vi "ZBX Control Example.vi"() -> ()   [LabVIEW 2023]
uses:
  <instrlib>/niUSRP/Reference FPGA/ZBX Control/ATR state.ctl
  <vilib>/Platform/TimedLoop/XDataNode/wakeup.ctl
  <vilib>/Platform/TimedLoop/XDataNode/XDNodeRunTimeDep.lvlib
  <vilib>/Platform/TimedLoop/XDataNode/nitl_modes.ctl
  <vilib>/Platform/TimedLoop/XDataNode/timing_clust.ctl
  <vilib>/Platform/TimedLoop/XDataNode/XDataNode.xnode
panel:
  in  "TX samples":u64
  in  "RX samples":u64
  in  "rx gain high":u32
  in  "rx gain low":u32
  in  "tx gain":u32
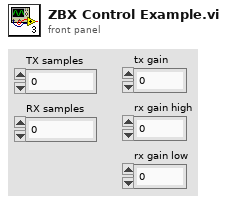
[diagram p1: front panel]
types:
  T1 = typedef "XDNodeRunTimeDep.lvlib/timing_clust.ctl" = cluster{"Expected End [f-1]":u64, "Actual End [f-1]":u64, "Finished Late? [f-1]":bool, "Expected End [i-1]":u64, "Actual End [i-1]":u64, "Finished Late? [i-1]":bool, "Expected Start [i]":u64, "Actual Start [i]":u64, "Expected Start [f]":u64, "Actual Start [f]":u64, "Source Name":string, "Structure Name":string, "Period":i64, "Deadline":i64, "Offset":i64, "Start":i64, "Priority":i32, "Timeout":i32, "Mode":T2, "Wakeup Reason":T3, "Error":errorcluster, "Source Type":string, "Secondary Source Type":string, "Global End Time":u64, "Global Start Time":u64, "Frame Duration":u64, "Iteration Duration":u64, "Assigned CPU":i32, "I/O Scan Engine Mode":u32}
  T2 = typedef "XDNodeRunTimeDep.lvlib/nitl_modes.ctl" = enum32{"No Change", "Process missed periods, maintain original phase", "Discard missed periods, maintain original phase", "Process missed periods, ignore original phase", "Discard missed periods, ignore original phase"}
  T3 = typedef "XDNodeRunTimeDep.lvlib/wakeup.ctl" = enum32{"Normal", "Aborted", "Asynchronous wakeup", "Timing source error", "Timed loop error", "Timeout"}
  T4 = typedef "ATR state.ctl" = enum8{"Idle", "RX", "TX", "TRX"}
  T5 = typedef "ZBX IO Response.ctl" = cluster{"response Ack":bool, "response data":u32, "response status":fxp<+,2,2>}
  T6 = typedef "ZBX IO Request.ctl" = cluster{"I/O Address":fxp<+,20,20>, "I/O Request Data":u32, "request write":bool, "request read":bool, "request has time":bool, "request time":u64}
  T7 = typedef "Dboard IOs.ctl" = cluster{"CtrlPortReqAddr":refnum<k21>, "CtrlPortReqData":refnum<k21>, "CtrlPortReqWr":refnum<k21>, "CtrlPortReqRd":refnum<k21>, "CtrlPortReqHasTime":refnum<k21>, "CtrlPortReqTime":refnum<k21>, "CtrlPortRespAck":refnum<k21>, "CtrlPortRespData":refnum<k21>, "CtrlPortRespStatus":refnum<k21>}
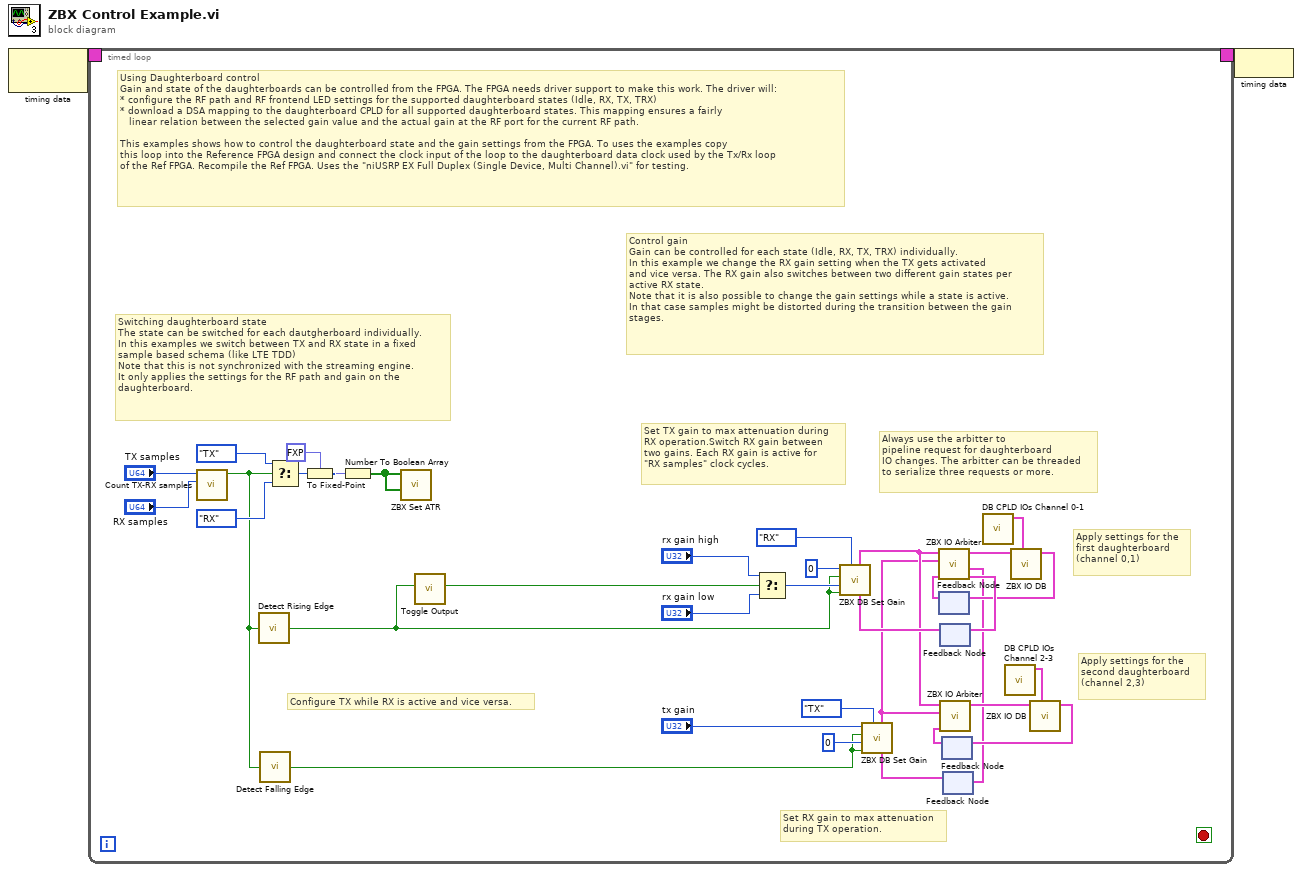
[diagram p0: block diagram]
diagram:
  n1 = node-c288() -> (w2:T1)  [unwired: 1 in]
  n2 = timed-loop {
    timing: w2 -> [_]
    timing-out: [_] -> w1
    stop <- _ stop-if-true
    # "Configure TX while RX is active and vice versa."
    # "Set RX gain to max attenuation\nduring TX operation."
    # "Set TX gain to max attenuation during\nRX operation.Switch RX gain between\ntwo gains. Each RX gain is active for\n\"RX samples\" clock cycles."
    # "Using Daughterboard control\nGain and state of the daughterboards can be controlled from the FPGA. The FPGA needs driver support to make this work. The driver will:\n* configure the RF path and RF frontend LED settings for the supported daughterboard states (Idle, RX, TX, TRX)\n* download a DSA mapping to the daughterboard CPLD for all supported daughterboard states. This mapping ensures a fairly \n   linear relation between the selected gain value and the actual gain at the RF port for the current RF path.\n\nThis examples shows how to control the daughterboard state and the gain settings from the FPGA. To uses the examples copy\nthis loop into the Reference FPGA design and connect the clock input of the loop to the daughterboard data clock used by the Tx/Rx loop\nof the Ref FPGA. Recompile the Ref FPGA. Uses the \"niUSRP EX Full Duplex (Single Device, Multi Channel).vi\" for testing."
    # "Always use the arbitter to\npipeline request for daughterboard\nIO changes. The arbitter can be threaded\nto serialize three requests or more."
    # "Apply settings for the\nsecond daughterboard \n(channel 2,3)"
    # "Apply settings for the\nfirst daughterboard \n(channel 0,1)"
    # "Control gain\nGain can be controlled for each state (Idle, RX, TX, TRX) individually.\nIn this example we change the RX gain setting when the TX gets activated\nand vice versa. The RX gain also switches between two different gain states per\nactive RX state.\nNote that it is also possible to change the gain settings while a state is active.\nIn that case samples might be distorted during the transition between the gain\nstages."
    # "Switching daughterboard state\nThe state can be switched for each dautgherboard individually.\nIn this examples we switch between TX and RX state in a fixed\nsample based schema (like LTE TDD)\nNote that this is not synchronized with the streaming engine. \nIt only applies the settings for the RF path and gain on the \ndaughterboard."
    n3 = call <instrlib>:"Count TX-RX samples.vi"("RX samples"="RX samples", "TX samples"="TX samples") -> ("is TX"=w5:bool)  [unwired: 8 in, 1 out]
    n4 = call <instrlib>:"Detect Rising Edge.vi"("signal"=w5) -> ("edge detected"=w6:bool)  [unwired: 14 in]
    n5 = call <instrlib>:"Detect Falling Edge.vi"("signal"=w5) -> ("edge detected"=w4:bool)  [unwired: 14 in]
    n6 = Select(t=ATR_state."TX" ("ATR state 2"), s=w5, f=ATR_state."RX") -> (s? t:f=w28:T4)
    n7 = To Fixed-Point(fixed-point type=fxp<+,4,4> 0.0, number=w28) -> (fixed-point=w27:fxp<+,4,4>)
    n8 = Number To Boolean Array(number=w27) -> (Boolean array=w25:bool[])
    n9 = call <instrlib>:"ZBX Set ATR.vi"("DB 1"=w25, "DB 0"=w25) -> ()  [unwired: 10 in]
    n10 = call <instrlib>:"Toggle Output.vi"("toggle"=w6) -> ("output"=w16:bool)  [unwired: 10 in]
    n11 = Select(t="rx gain high", s=w16, f="rx gain low") -> (s? t:f=w13:u32)
    n12 = feedback #1() -> (w36:T5)  [unwired: 1 in]
    n13 = feedback #2() -> (w23:T5)  [unwired: 1 in]
    n14 = call <instrlib>:"ZBX DB Set Gain.vi"("response in"=w23, "ATR state"=ATR_state."RX", "rx gain valid"=w6, "rx gain"=w13, "tx gain valid"=w6, "tx gain"=u32 0) -> ("request out"=w22:T6)  [unwired: 5 in]
    n15 = feedback #3() -> (w19:T5)  [unwired: 1 in]
    n16 = feedback #4() -> (w8:T5)  [unwired: 1 in]
    n17 = call <instrlib>:"ZBX DB Set Gain.vi"("response in"=w8, "ATR state"=ATR_state."TX", "rx gain valid"=w4, "rx gain"=u32 0, "tx gain valid"=w4, "tx gain"="tx gain") -> ("request out"=w7:T6)  [unwired: 5 in]
    n18 = call <instrlib>:"ZBX IO Arbiter.vi"("response"=w36, "request 2"=w7, "request 1"=w22) -> ("response 2"=w35:T5, "response1"=w9:T5, "request out"=w24:T6)  [unwired: 5 in, 1 out]
    n19 = feedback-in #2(w35) -> ()
    n20 = call <instrlib>:"ZBX IO Arbiter.vi"("response"=w19, "request 2"=w7, "request 1"=w22) -> ("request out"=w21:T6)  [unwired: 5 in, 3 out]
    n21 = feedback-in #4(w9) -> ()
    n22 = call <instrlib>:"DB CPLD IOs Channel 0-1.vi"() -> ("DBoard IOs"=w33:T7)  [unwired: 11 in]
    n23 = call <instrlib>:"DB CPLD IOs Channel 2-3.vi"() -> ("DBoard IOs"=w3:T7)  [unwired: 11 in]
    n24 = call <instrlib>:"ZBX IO DB.vi"("DBoard IOs"=w33, "request"=w24) -> ("response"=w34:T5)  [unwired: 9 in]
    n25 = feedback-in #1(w34) -> ()
    n26 = call <instrlib>:"ZBX IO DB.vi"("DBoard IOs"=w3, "request"=w21) -> ("response"=w20:T5)  [unwired: 9 in]
    n27 = feedback-in #3(w20) -> ()
  }
  n28 = node-c288(w1) -> ()
